vi "新数据.vi"(0 "Display State In":T1 caption="显示状态输入", 9 "Container State":T2 caption="容器状态", 11 "error in (no error)":errorcluster caption="错误输入（无错误）") -> (4 "Display State Out":T1 caption="显示状态输出", 15 "error out":errorcluster caption="错误输出")   [LabVIEW 2020, in "数据显示.xctl"]
uses:
  <vilib>/_xctls/Container State.ctl
  <vilib>/_xctls/XControlSupport.lvlib
panel:
  # "添加构成方法参数的输入控件及显示控件。连接至连线板。不要删除已连接至连线板的输入控件及显示控件。\n\n如需设置该方法的参数，右键单击项目树中的对应项并选择“配置方法...”。"
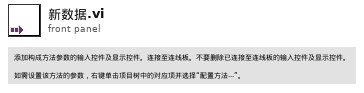
[diagram p1: front panel]
types:
  T1 = typedef "数据显示.xctl/状态.ctl" = cluster{"历史数据":cluster{"数组":dbl[][]}[], "数据":dbl[][], "保留数量":i32, "完成":bool, "扫描":bool}
  T2 = typedef "XControlSupport.lvlib/Container State.ctl" = cluster{"Indicator?":bool, "Run Mode?":bool, " Refnum":refnum<vi>}
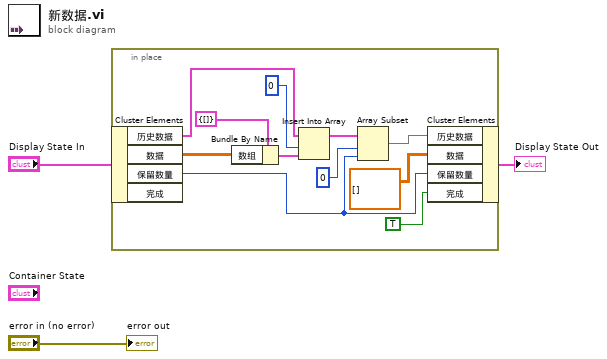
[diagram p0: block diagram]
diagram:
  n1 = in-place {
    n2 = in-place-cluster #1("Display State In") -> ("历史数据"=w14:cluster{"数组":dbl[][]}[], "数据"=w11:dbl[][], "保留数量"=w6:i32)  [unwired: 1 out]
    n3 = Bundle By Name(cluster=cluster{"数组":dbl[][]} {"数组"=[]} ("新元素/子数组"), "数组"=w11) -> (w12:cluster{"数组":dbl[][]})
    n4 = Insert Into Array(array=w14, index=0 ("索引"), new element=w12) -> (w8:cluster{"数组":dbl[][]}[])
    n5 = Array Subset(array=w8, index=0 ("索引"), length=w6) -> (w5:cluster{"数组":dbl[][]}[])
    n6 = in-place-cluster #1("历史数据"=w5, "数据"=dbl[][] [], "保留数量"=w6, "完成"=TRUE) -> (→"Display State Out":T1)
  }
  "error out" <- "error in (no error)"
